vi "ExMove3Spectro.vi"() -> ()   [LabVIEW 2010]
panel:
  in  "Grating number 3":i16=1 min=1 max=100 step=1
  in  "Grating Speed 3":dbl=2000.0 min=1.0 step=1.0 format="%.2f"
  in  "Start Wavelength 3":dbl format="%.2f"
  in  "End Wavelength 3":dbl=700.0 format="%.2f"
  in  "Increment Wavelength 3":dbl=50.0 format="%.2f"
  out "Current Wavelength 3":string
  out "error out 3":errorcluster
  out "error out 2":errorcluster
  out "Current Wavelength 2":string
  in  "Increment Wavelength 2":dbl=50.0 format="%.2f"
  in  "End Wavelength 2":dbl=700.0 format="%.2f"
  in  "Start Wavelength 2":dbl format="%.2f"
  in  "Grating Speed 2":dbl=2000.0 min=1.0 step=1.0 format="%.2f"
  in  "Grating number 2":i16=1 min=1 max=100 step=1
  out "Current Wavelength":string
  in  "Increment Wavelength":dbl=50.0 format="%.2f"
  in  "End Wavelength":dbl=700.0 format="%.2f"
  in  "Start Wavelength":dbl format="%.2f"
  in  "Grating Speed":dbl=2000.0 min=1.0 step=1.0 format="%.2f"
  in  "Grating number":i16=1 min=1 max=100 step=1
  out "error out":errorcluster
  in  "error in (no error)":errorcluster
  # "NOTES:\nA properly configured spectometer .ini must be present in the LabVIEW folder for spectrograph operation.  This MUST be defined for 3 spectrographs.\n\nConsult the Toolkit documentation for more information on how to configure this file."
  # "ExMove3Spectro.vi\n(Normal Spectrograph via USB/COM port)\nThis VI is a simple example of how to setup and move 3 spectrographs in increments over a wavelength range."
  # "SPECTROGRAPH 3"
  # "SPECTROGRAPH 2"
  # "SPECTROGRAPH 1"
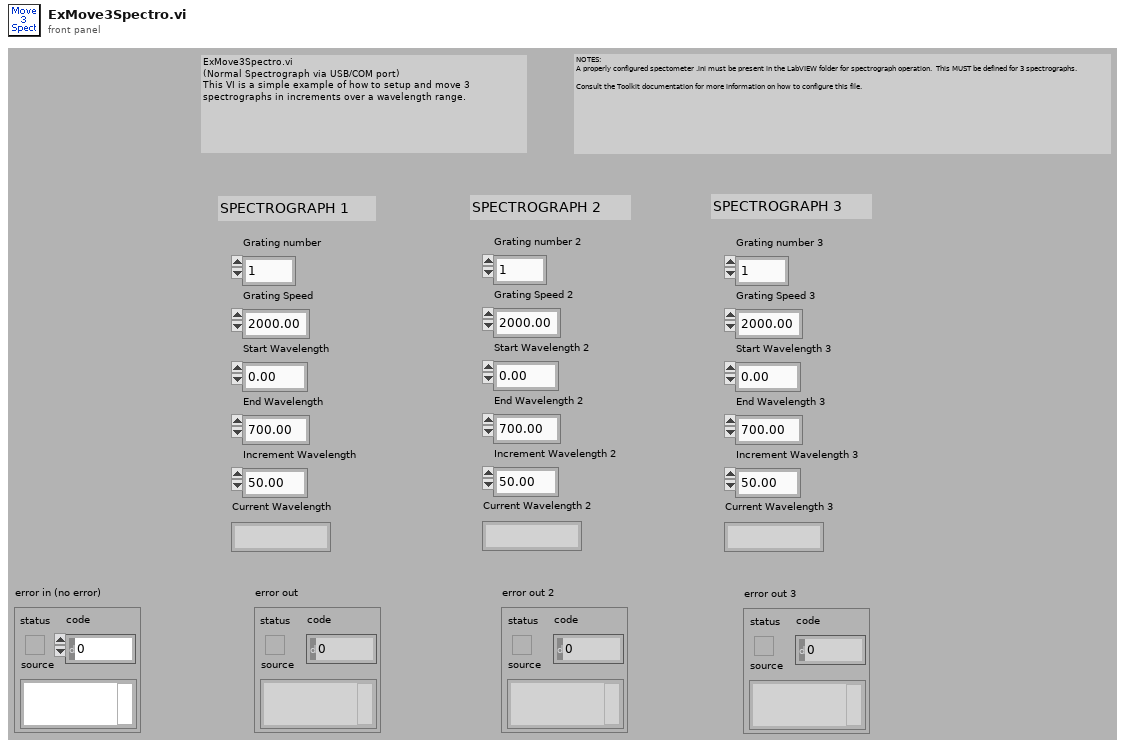
[diagram p1: front panel]
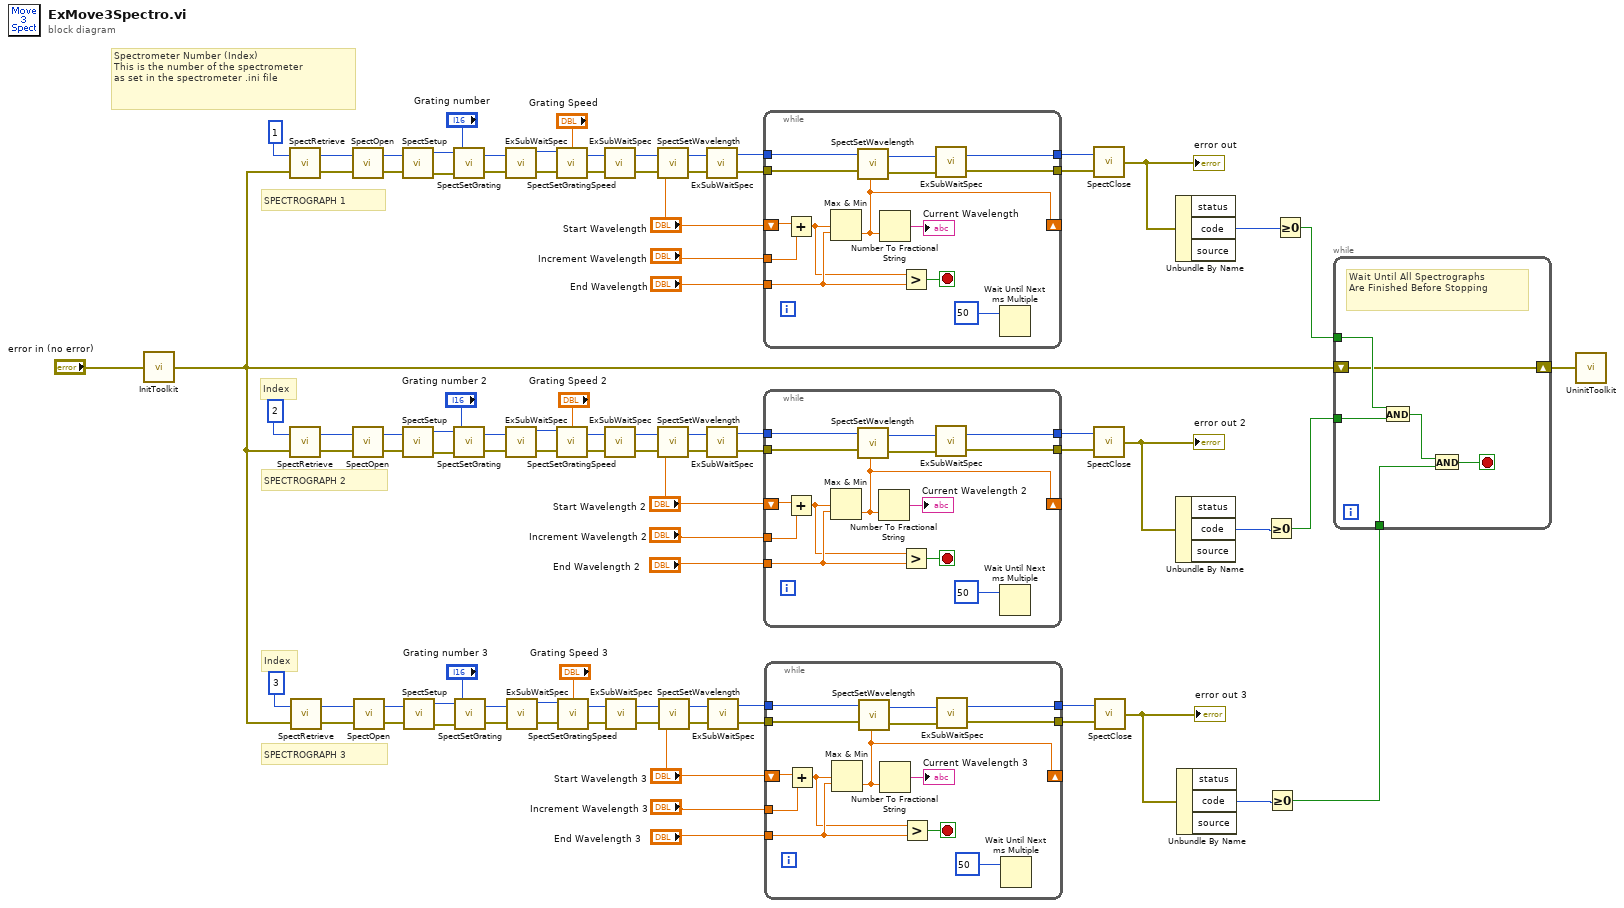
[diagram p0: block diagram]
diagram:
  # "SPECTROGRAPH 3"
  # "SPECTROGRAPH 2"
  # "SPECTROGRAPH 1"
  # "Index"
  # "Index"
  # "Spectrometer Number (Index)\nThis is the number of the spectrometer\nas set in the spectrometer .ini file"
  n1 = call <userlib>:"InitToolkit.vi"("error in"="error in (no error)") -> ("error out"=w2:errorcluster)
  n2 = call <userlib>:"SpectRetrieve.vi"("error in"=w2, "Index"=1) -> ("error out"=w68:errorcluster, "Device ID"=w67:u32)
  n3 = call <userlib>:"SpectRetrieve.vi"("error in"=w2, "Index"=2) -> ("error out"=w49:errorcluster, "Device ID"=w48:u32)
  n4 = call <userlib>:"SpectRetrieve.vi"("error in"=w2, "Index"=3) -> ("error out"=w16:errorcluster, "Device ID"=w15:u32)
  n5 = call <userlib>:"SpectOpen.vi"("error in"=w68, "Spectrometer ID"=w67) -> ("error out"=w72:errorcluster, "Spectrometer Handle"=w74:u32)  [unwired: 1 in]
  n6 = call <userlib>:"SpectOpen.vi"("error in"=w49, "Spectrometer ID"=w48) -> ("error out"=w51:errorcluster, "Spectrometer Handle"=w53:u32)  [unwired: 1 in]
  n7 = call <userlib>:"SpectOpen.vi"("error in"=w16, "Spectrometer ID"=w15) -> ("error out"=w18:errorcluster, "Spectrometer Handle"=w20:u32)  [unwired: 1 in]
  n8 = call <userlib>:"SpectSetup.vi"("error in"=w72, "Spectrometer Handle"=w74) -> ("error out"=w71:errorcluster, "Spectrometer Handle"=w73:u32)
  n9 = call <userlib>:"SpectSetup.vi"("error in"=w51, "Spectrometer Handle"=w53) -> ("error out"=w50:errorcluster, "Spectrometer Handle"=w52:u32)
  n10 = call <userlib>:"SpectSetup.vi"("error in"=w18, "Spectrometer Handle"=w20) -> ("error out"=w17:errorcluster, "Spectrometer Handle"=w19:u32)
  n11 = call <userlib>:"SpectSetGrating.vi"("error in"=w71, "Grating Number"="Grating number", "Sepctrometer Handle"=w73) -> ("error out"=w80:errorcluster, "Spectrometer Handle"=w79:u32)
  n12 = call <userlib>:"SpectSetGrating.vi"("error in"=w50, "Grating Number"="Grating number 2", "Sepctrometer Handle"=w52) -> ("error out"=w59:errorcluster, "Spectrometer Handle"=w58:u32)
  n13 = call <userlib>:"SpectSetGrating.vi"("error in"=w17, "Grating Number"="Grating number 3", "Sepctrometer Handle"=w19) -> ("error out"=w26:errorcluster, "Spectrometer Handle"=w25:u32)
  n14 = call "ExSubWaitSpec.vi"("error in (no error)"=w80, "Spectrometer Handle"=w79) -> ("error out"=w78:errorcluster, "Spectrometer handle"=w77:u32)
  n15 = call "ExSubWaitSpec.vi"("error in (no error)"=w59, "Spectrometer Handle"=w58) -> ("error out"=w57:errorcluster, "Spectrometer handle"=w56:u32)
  n16 = call "ExSubWaitSpec.vi"("error in (no error)"=w26, "Spectrometer Handle"=w25) -> ("error out"=w24:errorcluster, "Spectrometer handle"=w23:u32)
  n17 = call <userlib>:"SpectSetGratingSpeed.vi"("error in"=w78, "Grating Speed"="Grating Speed", "Spectrometer Handle"=w77) -> ("error out"=w75:errorcluster, "Spectrometer Handle"=w76:u32)
  n18 = call <userlib>:"SpectSetGratingSpeed.vi"("error in"=w57, "Grating Speed"="Grating Speed 2", "Spectrometer Handle"=w56) -> ("error out"=w54:errorcluster, "Spectrometer Handle"=w55:u32)
  n19 = call <userlib>:"SpectSetGratingSpeed.vi"("error in"=w24, "Grating Speed"="Grating Speed 3", "Spectrometer Handle"=w23) -> ("error out"=w21:errorcluster, "Spectrometer Handle"=w22:u32)
  n20 = call "ExSubWaitSpec.vi"("error in (no error)"=w75, "Spectrometer Handle"=w76) -> ("error out"=w65:errorcluster, "Spectrometer handle"=w66:u32)
  n21 = call "ExSubWaitSpec.vi"("error in (no error)"=w54, "Spectrometer Handle"=w55) -> ("error out"=w46:errorcluster, "Spectrometer handle"=w47:u32)
  n22 = call "ExSubWaitSpec.vi"("error in (no error)"=w21, "Spectrometer Handle"=w22) -> ("error out"=w13:errorcluster, "Spectrometer handle"=w14:u32)
  n23 = call <userlib>:"SpectSetWavelength.vi"("error in"=w65, "Wavelength"="Start Wavelength", "Spectrometer Handle"=w66) -> ("error out"=w90:errorcluster, "Spectrumeter Handle"=w89:u32)
  n24 = call <userlib>:"SpectSetWavelength.vi"("error in"=w46, "Wavelength"="Start Wavelength 2", "Spectrometer Handle"=w47) -> ("error out"=w63:errorcluster, "Spectrumeter Handle"=w62:u32)
  n25 = call <userlib>:"SpectSetWavelength.vi"("error in"=w13, "Wavelength"="Start Wavelength 3", "Spectrometer Handle"=w14) -> ("error out"=w30:errorcluster, "Spectrumeter Handle"=w29:u32)
  n26 = call "ExSubWaitSpec.vi"("error in (no error)"=w90, "Spectrometer Handle"=w89) -> ("error out"=w82:errorcluster, "Spectrometer handle"=w88:u32)
  n27 = call "ExSubWaitSpec.vi"("error in (no error)"=w63, "Spectrometer Handle"=w62) -> ("error out"=w60:errorcluster, "Spectrometer handle"=w61:u32)
  n28 = call "ExSubWaitSpec.vi"("error in (no error)"=w30, "Spectrometer Handle"=w29) -> ("error out"=w27:errorcluster, "Spectrometer handle"=w28:u32)
  n29 = while {
    tunnel: w88 -> [w95]
    tunnel: "Increment Wavelength" -> [w102]
    tunnel: "End Wavelength" -> [w94]
    shift-right: [w92] -> _
    shift-left: "Start Wavelength" -> [w103]
    tunnel: [w99] -> w84
    tunnel: [w96] -> w83
    tunnel: w82 -> [w98]
    stop <- w93 stop-if-true
    n30 = Add(x=w103, y=w102) -> (x+y=w91:dbl)
    n31 = Max & Min(x=w91, y=w94) -> (min(x,y)=w92:dbl)  [unwired: 1 out]
    n32 = call <userlib>:"SpectSetWavelength.vi"("error in"=w98, "Wavelength"=w92, "Spectrometer Handle"=w95) -> ("error out"=w97:errorcluster, "Spectrumeter Handle"=w100:u32)
    n33 = Number To Fractional String(number=w92) -> (F-format string=→"Current Wavelength":string)  [unwired: 3 in]
    n34 = Greater?(x=w91, y=w94) -> (0:w93:bool)
    n35 = call "ExSubWaitSpec.vi"("error in (no error)"=w97, "Spectrometer Handle"=w100) -> ("error out"=w96:errorcluster, "Spectrometer handle"=w99:u32)
    n36 = Wait Until Next ms Multiple(millisecond multiple=50) -> ()  [unwired: 1 out]
  }
  n37 = while {
    tunnel: w61 -> [w110]
    tunnel: "Increment Wavelength 2" -> [w116]
    tunnel: "End Wavelength 2" -> [w109]
    shift-right: [w107] -> _
    shift-left: "Start Wavelength 2" -> [w117]
    tunnel: [w114] -> w39
    tunnel: [w111] -> w38
    tunnel: w60 -> [w113]
    stop <- w108 stop-if-true
    n38 = Add(x=w117, y=w116) -> (x+y=w106:dbl)
    n39 = Max & Min(x=w106, y=w109) -> (min(x,y)=w107:dbl)  [unwired: 1 out]
    n40 = call <userlib>:"SpectSetWavelength.vi"("error in"=w113, "Wavelength"=w107, "Spectrometer Handle"=w110) -> ("error out"=w112:errorcluster, "Spectrumeter Handle"=w115:u32)
    n41 = Number To Fractional String(number=w107) -> (F-format string=→"Current Wavelength 2":string)  [unwired: 3 in]
    n42 = Greater?(x=w106, y=w109) -> (0:w108:bool)
    n43 = call "ExSubWaitSpec.vi"("error in (no error)"=w112, "Spectrometer Handle"=w115) -> ("error out"=w111:errorcluster, "Spectrometer handle"=w114:u32)
    n44 = Wait Until Next ms Multiple(millisecond multiple=50) -> ()  [unwired: 1 out]
  }
  n45 = while {
    tunnel: w28 -> [w124]
    tunnel: "Increment Wavelength 3" -> [w130]
    tunnel: "End Wavelength 3" -> [w123]
    shift-right: [w121] -> _
    shift-left: "Start Wavelength 3" -> [w131]
    tunnel: [w128] -> w6
    tunnel: [w125] -> w5
    tunnel: w27 -> [w127]
    stop <- w122 stop-if-true
    n46 = Add(x=w131, y=w130) -> (x+y=w120:dbl)
    n47 = Max & Min(x=w120, y=w123) -> (min(x,y)=w121:dbl)  [unwired: 1 out]
    n48 = call <userlib>:"SpectSetWavelength.vi"("error in"=w127, "Wavelength"=w121, "Spectrometer Handle"=w124) -> ("error out"=w126:errorcluster, "Spectrumeter Handle"=w129:u32)
    n49 = Number To Fractional String(number=w121) -> (F-format string=→"Current Wavelength 3":string)  [unwired: 3 in]
    n50 = Greater?(x=w120, y=w123) -> (0:w122:bool)
    n51 = call "ExSubWaitSpec.vi"("error in (no error)"=w126, "Spectrometer Handle"=w129) -> ("error out"=w125:errorcluster, "Spectrometer handle"=w128:u32)
    n52 = Wait Until Next ms Multiple(millisecond multiple=50) -> ()  [unwired: 1 out]
  }
  n53 = call <userlib>:"SpectClose.vi"("error in"=w83, "Spectrometer Handle"=w84) -> ("error out"=w37:errorcluster)
  "error out" <- w37
  n54 = call <userlib>:"SpectClose.vi"("error in"=w38, "Spectrometer Handle"=w39) -> ("error out"=w33:errorcluster)
  "error out 2" <- w33
  n55 = call <userlib>:"SpectClose.vi"("error in"=w5, "Spectrometer Handle"=w6) -> ("error out"=w4:errorcluster)
  "error out 3" <- w4
  n56 = Unbundle By Name(w37) -> ("code"=w36:i32)  [unwired: 2 out]
  n57 = Unbundle By Name(w33) -> ("code"=w32:i32)  [unwired: 2 out]
  n58 = Unbundle By Name(w4) -> ("code"=w3:i32)  [unwired: 2 out]
  n59 = Greater Or Equal To 0?(x=w32) -> (x >= 0?=w31:bool)
  n60 = Greater Or Equal To 0?(x=w3) -> (x >= 0?=w1:bool)
  n61 = Greater Or Equal To 0?(x=w36) -> (x >= 0?=w34:bool)
  n62 = while {
    shift-right: [w136] -> w35
    shift-left: w2 -> [w136]
    tunnel: w34 -> [w138]
    tunnel: w31 -> [w137]
    tunnel: w1 -> [w135]
    stop <- w133 stop-if-true
    # "Wait Until All Spectrographs\nAre Finished Before Stopping"
    n63 = And(x=w138, y=w137) -> (x .and. y?=w134:bool)
    n64 = And(x=w134, y=w135) -> (x .and. y?=w133:bool)
  }
  n65 = call <userlib>:"UninitToolkit.vi"("error in"=w35) -> ()  [unwired: 1 out]
